vi "Save NG Result.vi"(7 "Table":refnum<vi>, 8 "error in (no error)":errorcluster, 10 "ProductID":string, 11 "strXMLResultText":string) -> (0 "error out":errorcluster, 1 "结果字符串":string, 2 "Error Code":i64, 3 "Operation Success":bool)   [LabVIEW 2017]
panel:
  in  "FFTester._Tester":refnum<k7>
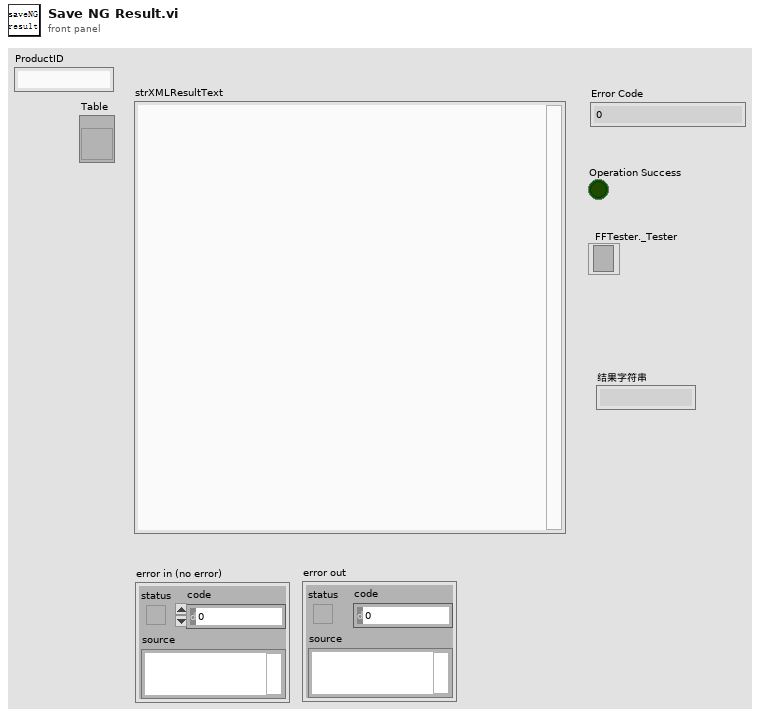
[diagram p1: front panel]
types:
  T1 = enum16{"open", "replace", "create", "open or create", "replace or create", "replace or create with confirmation"}
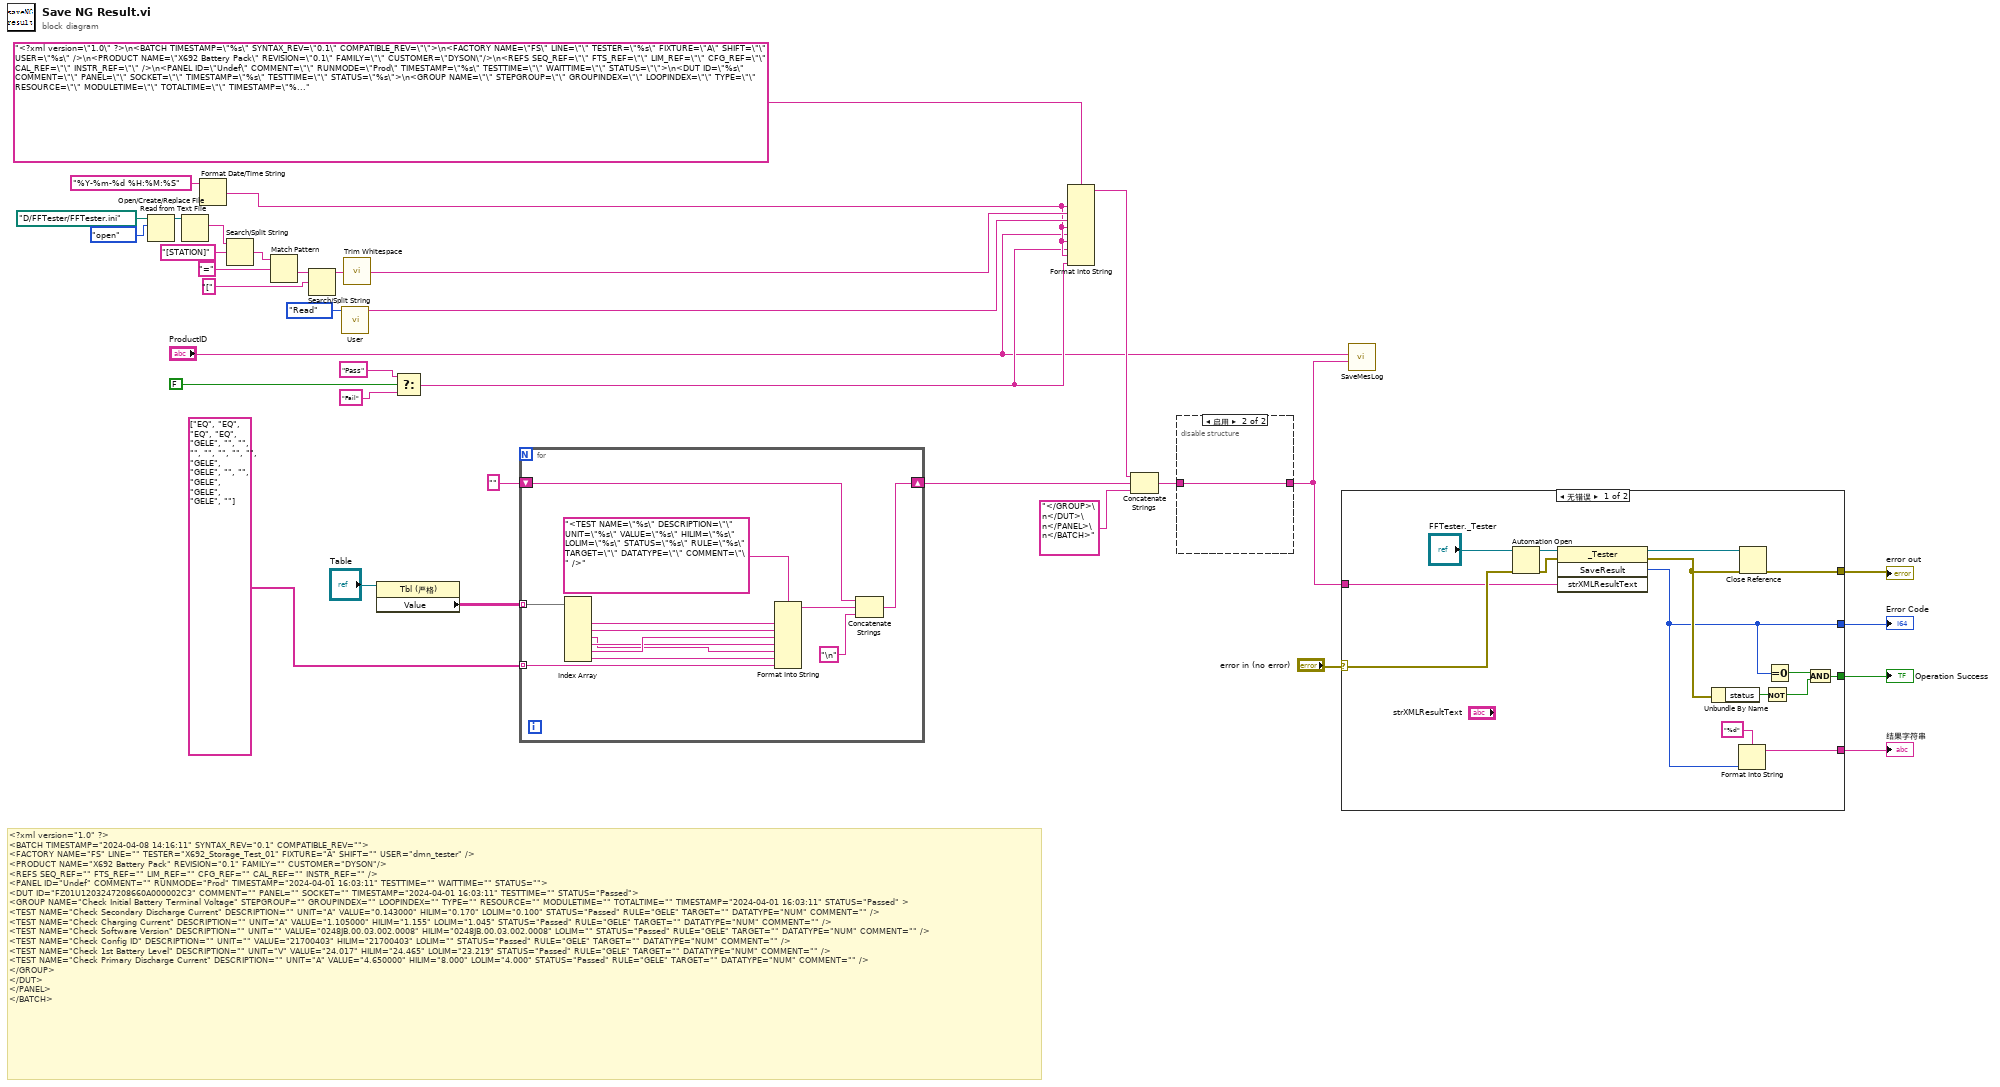
[diagram p0: block diagram]
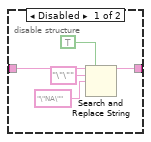
[diagram p2: hidden frame]
diagram:
  # "<?xml version=\"1.0\" ?>\n<BATCH TIMESTAMP=\"2024-04-08 14:16:11\" SYNTAX_REV=\"0.1\" COMPATIBLE_REV=\"\">\n<FACTORY NAME=\"FS\" LINE=\"\" TESTER=\"X692_Storage_Test_01\" FIXTURE=\"A\" SHIFT=\"\" USER=\"dmn_tester\" />\n<PRODUCT NAME=\"X692 Battery Pack\" REVISION=\"0.1\" FAMILY=\"\" CUSTOMER=\"DYSON\"/>\n<REFS SEQ_REF=\"\" FTS_REF=\"\" LIM_REF=\"\" CFG_REF=\"\" CAL_REF=\"\" INSTR_REF=\"\" />\n<PANEL ID=\"Undef\" COMMENT=\"\" RUNMODE=\"Prod\" TIMESTAMP=\"2024-04-01 16:03:11\" TESTTIME=\"\" WAITTIME=\"\" STATUS=\"\">\n<DUT ID=\"FZ01U1203247208660A000002C3\" COMMENT=\"\" PANEL=\"\" SOCKET=\"\" TIMESTAMP=\"2024-04-01 16:03:11\" TESTTIME=\"\" STATUS=\"Passed\">\n<GROUP NAME=\"Check Initial Battery Terminal Voltage\" STEPGROUP=\"\" GROUPINDEX=\"\" LOOPINDEX=\"\" TYPE=\"\" RESOURCE=\"\" MODULETIME=\"\" TOTALTIME=\"\" TIMESTAMP=\"2024-04-01 16:03:11\" STATUS=\"Passed\" >\n<TEST NAME=\"Check Secondary Discharge Current\" DESCRIPTION=\"\" UNIT=\"A\" VALUE=\"0.143000\" HILIM=\"0.170\" LOLIM=\"0.100\" STATUS=\"Passed\" RULE=\"GELE\" TARGET=\"\" DATATYPE=\"NUM\" COMMENT=\"\" />\n<TEST NAME=\"Check Charging Current\" DESCRIPTION=\"\" UNIT=\"A\" VALUE=\"1.105000\" HILIM=\"1.155\" LOLIM=\"1.045\" STATUS=\"Passed\" RULE=\"GELE\" TARGET=\"\" DATATYPE=\"NUM\" COMMENT=\"\" />\n<TEST NAME=\"Check Software Version\" DESCRIPTION=\"\" UNIT=\"\" VALUE=\"0248JB.00.03.002.0008\" HILIM=\"0248JB.00.03.002.0008\" LOLIM=\"\" STATUS=\"Passed\" RULE=\"GELE\" TARGET=\"\" DATATYPE=\"NUM\" COMMENT=\"\" />\n<TEST NAME=\"Check Config ID\" DESCRIPTION=\"\" UNIT=\"\" VALUE=\"21700403\" HILIM=\"21700403\" LOLIM=\"\" STATUS=\"Passed\" RULE=\"GELE\" TARGET=\"\" DATATYPE=\"NUM\" COMMENT=\"\" />\n<TEST NAME=\"Check 1st Battery Level\" DESCRIPTION=\"\" UNIT=\"V\" VALUE=\"24.017\" HILIM=\"24.465\" LOLIM=\"23.219\" STATUS=\"Passed\" RULE=\"GELE\" TARGET=\"\" DATATYPE=\"NUM\" COMMENT=\"\" />\n<TEST NAME=\"Check Primary Discharge Current\" DESCRIPTION=\"\" UNIT=\"A\" VALUE=\"4.650000\" HILIM=\"8.000\" LOLIM=\"4.000\" STATUS=\"Passed\" RULE=\"GELE\" TARGET=\"\" DATATYPE=\"NUM\" COMMENT=\"\" />\n</GROUP>\n</DUT>\n</PANEL>\n</BATCH>"
  n1 = Open/Create/Replace File(file path (use dialog)=path "D:/FFTester/FFTester.ini" ("路径"), operation (0:open)=T1."open" ("操作(0:open)")) -> (refnum out=w17:refnum<file>)  [unwired: 4 in, 2 out]
  n2 = Read from Text File(file (use dialog)=w17) -> (text=w18:string)  [unwired: 3 in, 3 out]
  n3 = Format Date/Time String(time format string (%c)="%Y-%m-%d %H:%M:%S" ("时间格式字符串(%c)")) -> (date/time string=w6:string)  [unwired: 2 in]
  n4 = Search/Split String(string=w18, search string/char (-)="[STATION]") -> (match + rest of string=w19:string)  [unwired: 1 in, 2 out]
  n5 = Match Pattern(string=w19, regular expression="=") -> (after substring=w21:string)  [unwired: 1 in, 3 out]
  n6 = Search/Split String(string=w21, search string/char (-)="[") -> (substring before match=w20:string)  [unwired: 1 in, 2 out]
  n7 = call "User.vi"("Step"=enum16{"Initial", "Write", "Read"}."Read") -> ("User out"=w9:string)  [unwired: 9 in, 1 out]
  n8 = call <vilib>:"Trim Whitespace.vi"("string"=w20) -> ("trimmed string"=w11:string)  [unwired: 1 in]
  n9 = property class="Tbl (严格)"(reference="Table") -> ("Value"=w30:string[][])  [unwired: 1 in, 2 out]
  n10 = Select(t="Pass", s=FALSE, f="Fail") -> (s? t:f=w5:string)
  n11 = for {
    tunnel: w30 -> [w48] mode=indexing
    tunnel: string[] ["EQ", "EQ", "EQ", "EQ", "GELE", "", "", "", "", "", "", "", "GELE", "GELE", "", "", "GELE", "GELE", "GELE", ""] -> [w40] mode=indexing
    shift-right: [w36] -> w27
    shift-left: "" -> [w37]
    n12 = Index Array(array=w48) -> (element #2=w46:string, element #3=w45:string, element #4=w42:string, element #5=w43:string, element #6=w44:string, element #7=w41:string)  [unwired: 7 in, 1 out]
    n13 = Format Into String(format string="<TEST NAME=\"%s\" DESCRIPTION=\"\" UNIT=\"%s\" VALUE=\"%s\" HILIM=\"%s\" LOLIM=\"%s\" STATUS=\"%s\" RULE=\"%s\" TARGET=\"\" DATATYPE=\"\" COMMENT=\"\" />", w46, w45, w44, w43, w42, w41, w40) -> (resulting string=w39:string)  [unwired: 2 in, 1 out]
    n14 = Concatenate Strings(w37, w39, "\n") -> (w36:string)
  }
  n15 = Format Into String(format string="<?xml version=\"1.0\" ?>\n<BATCH TIMESTAMP=\"%s\" SYNTAX_REV=\"0.1\" COMPATIBLE_REV=\"\">\n<FACTORY NAME=\"FS\" LINE=\"\" TESTER=\"%s\" FIXTURE=\"A\" SHIFT=\"\" USER=\"%s\" />\n<PRODUCT NAME=\"X692 Battery Pack\" REVISION=\"0.1\" FAMILY=\"\" CUSTOMER=\"DYSON\"/>\n<REFS SEQ_REF=\"\" FTS_REF=\"\" LIM_REF=\"\" CFG_REF=\"\" CAL_REF=\"\" INSTR_REF=\"\" />\n<PANEL ID=\"Undef\" COMMENT=\"\" RUNMODE=\"Prod\" TIMESTAMP=\"%s\" TESTTIME=\"\" WAITTIME=\"\" STATUS=\"\">\n<DUT ID=\"%s\" COMMENT=\"\" PANEL=\"\" SOCKET=\"\" TIMESTAMP=\"%s\" TESTTIME=\"\" STATUS=\"%s\">\n<GROUP NAME=\"\" STEPGROUP=\"\" GROUPINDEX=\"\" LOOPINDEX=\"\" TYPE=\"\" RESOURCE=\"\" MODULETIME=\"\" TOTALTIME=\"\" TIMESTAMP=\"%s\" STATUS=\"%s\" >\n", w6, w11, w9, w6, "ProductID", w6, w5, w6, w5) -> (resulting string=w23:string)  [unwired: 2 in, 1 out]
  n16 = Concatenate Strings(w23, w27, "</GROUP>\n</DUT>\n</PANEL>\n</BATCH>") -> (w22:string)
  n17 = disable-structure shown="启用" {
    disable-tunnel: [w53 w54] -> w1
    disable-tunnel: w22 -> [w52 w54]
    frame Disabled {
      n18 = Search and Replace String(replace all?=TRUE ("替换全部？(F)"), input string=w52, search string="\"\"" ("搜索字符串"), replace string="\"NA\"" ("搜索字符串")) -> (result string=w53:string)  [unwired: 4 in, 3 out]
    }
    frame Enabled {
    }
  }
  n19 = case shown="无错误" "error in (no error)" {
    selector: "error in (no error)" -> [w62 w70]
    tunnel: [w69 w70] -> w35
    tunnel: [w56 _] -> w33
    tunnel: [w65 _] -> w32
    tunnel: w1 -> [w58 _]
    tunnel: [w55 _] -> w4
    frame No Error {
      n20 = Automation Open(error in (no error)=w62, Automation Refnum="FFTester._Tester") -> (Automation Refnum=w64:refnum<k7>, error out=w61:errorcluster)  [unwired: 2 in]
      n21 = invoke on="调用节点" class="_Tester" method="SaveResult"(reference=w64, error in=w61, "strXMLResultText"=w58) -> (reference out=w59:refnum<k7>, error out=w60:errorcluster, "SaveResult"=w56:i32)  [unwired: 1 in, 1 out]
      n22 = Unbundle By Name(w60) -> ("status"=w68:bool)
      n23 = Format Into String(format string="%d" ("格式字符串"), w56) -> (resulting string=w55:string)  [unwired: 2 in, 1 out]
      n24 = Close Reference(reference=w59, error in (no error)=w60) -> (error out=w69:errorcluster)
      n25 = Not(x=w68) -> (.not. x?=w66:bool)
      n26 = Equal To 0?(x=w56) -> (x = 0?=w67:bool)
      n27 = And(x=w67, y=w66) -> (x .and. y?=w65:bool)
    }
    frame Error {
    }
  }
  "error out" <- w35
  "Error Code" <- w33
  "Operation Success" <- w32
  "结果字符串" <- w4
  n28 = call "SaveMesLog.vi"("String"=w1, "SN"="ProductID") -> ()  [unwired: 10 in]
